vi "rvc Generate Multi-dimensional trajectory.vi"(6 "type of interpolator":u16(ring) items=["polynomial", "Linear with Blend"], 9 "number of timesteps":dbl, 10 "final position array":dbl[](array[numeric]), 11 "initial position array":dbl[](array[numeric])) -> (0 "error out":errorcluster, 1 "multi-segment trajectories":dbl[][](array[numeric]), 2 "time":dbl[](array[numeric]), 3 "position":cluster{dbl[], "P(A)":dbl[]}[](graph))   [LabVIEW 2017]
doc: "mtraj"
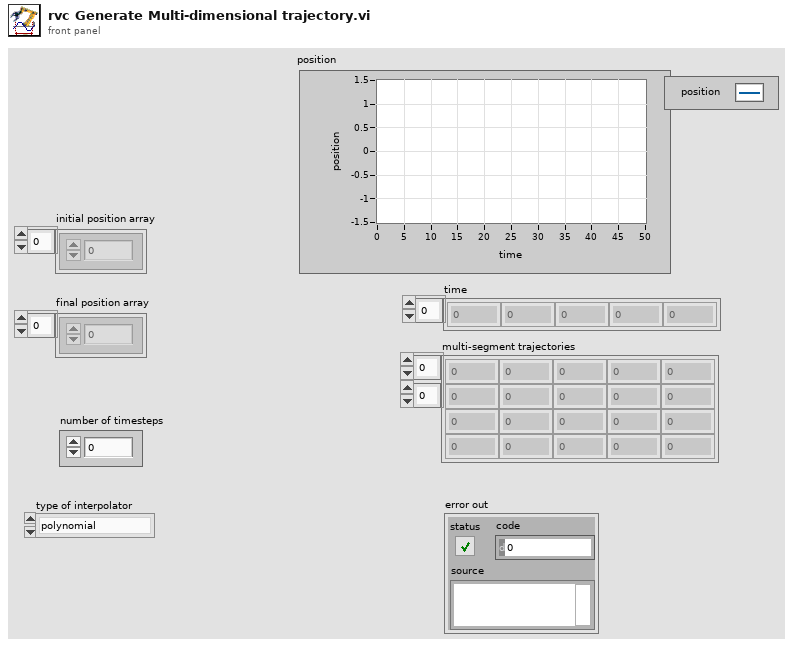
[diagram p1: front panel]
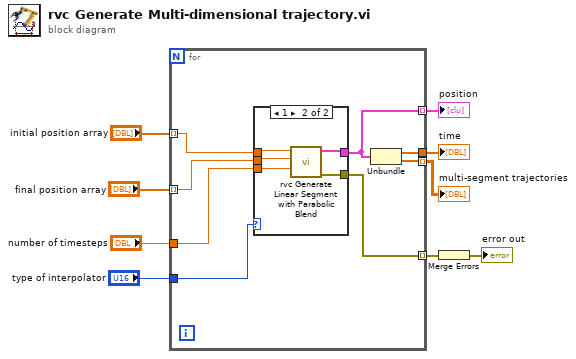
[diagram p0: block diagram]
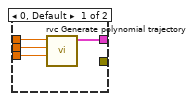
[diagram p2: hidden frame]
diagram:
  n1 = for {
    tunnel: "initial position array" -> [w17] mode=indexing
    tunnel: "final position array" -> [w16] mode=indexing
    tunnel: "number of timesteps" -> [w15]
    tunnel: "type of interpolator" -> [w14]
    tunnel: [w13] -> w4 mode=indexing
    tunnel: [w12] -> w5
    tunnel: [w11] -> w3 mode=indexing
    tunnel: [w10] -> w2 mode=indexing
    n2 = case shown="1" w14 {
      tunnel: [w21 w23] -> w11
      tunnel: w17 -> [w20 w26]
      tunnel: w16 -> [w19 w25]
      tunnel: w15 -> [w18 w24]
      tunnel: [_ w22] -> w10
      frame 0, Default {
        n3 = call "rvc Generate polynomial trajectory.vi"("number of timesteps"=w18, "final position"=w19, "initial position"=w20) -> ("position"=w21:cluster{"time":dbl[], "position":dbl[]})  [unwired: 6 in, 2 out]
      }
      frame 1 {
        n4 = call "rvc Generate Linear Segment with Parabolic Blend.vi"("number of timesteps"=w24, "final position"=w25, "initial position"=w26) -> ("error out"=w22:errorcluster, "position"=w23:cluster{"time":dbl[], "position":dbl[]})  [unwired: 5 in, 2 out]
      }
    }
    n5 = Unbundle(w11) -> ("time"=w12:dbl[], "position"=w13:dbl[])
  }
  "time" <- w5
  "multi-segment trajectories" <- w4
  "position" <- w3
  n6 = Merge Errors(w2) -> (→"error out":errorcluster)
